vi "Update GEA FGV.vi"(8 "Error In":errorcluster, 10 "Enum":enum16{"Read", "Write"}(ring), 11 "GEA Inputs":T1 {"Destination" format="%.0x"; "Source" format="%.0x"}) -> (0 "Error Out":errorcluster, 3 "GEA Out":T1[](array[typedef]) {"Destination" format="%.0x"; "Source" format="%.0x"})   [LabVIEW 2016]
uses:
  Common/LabVIEW GEA2 Toolkit/LabVIEW_GEA2_Toolkit.lvlibp/type defs/Source_Destination.ctl
  Common/LabVIEW GEA2 Toolkit/LabVIEW_GEA2_Toolkit.lvlibp
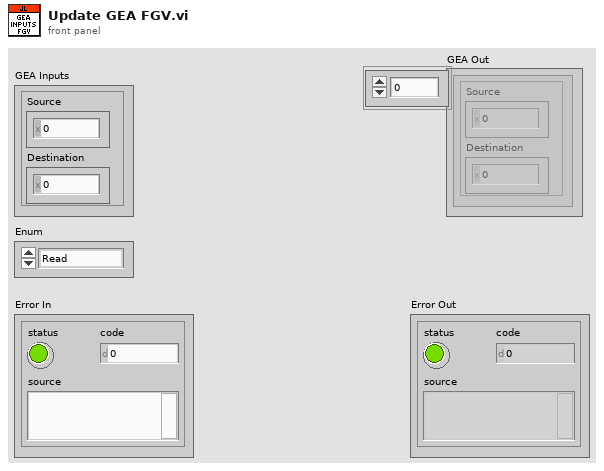
[diagram p1: front panel]
types:
  T1 = typedef "LabVIEW_GEA2_Toolkit.lvlibp/Source_Destination.ctl" = cluster{"Source":u8, "Destination":u8}
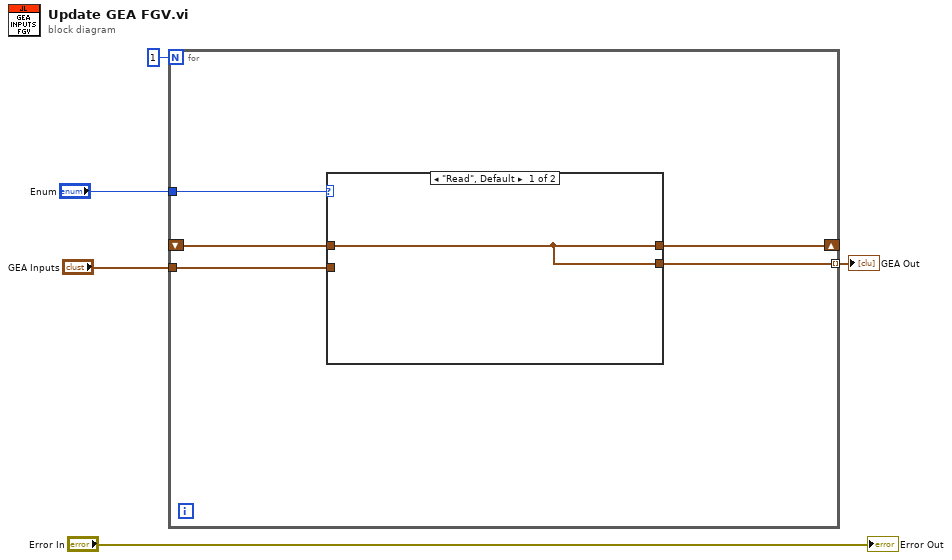
[diagram p0: block diagram]
diagram:
  n1 = for {
    N: 1 -> [_]
    shift-right: [w7] -> _
    shift-left: _ -> [w10]
    tunnel: "GEA Inputs" -> [w9]
    tunnel: "Enum" -> [w8]
    tunnel: [w6] -> w2 mode=indexing
    n2 = case shown="\"Read\", Default" w8 {
      tunnel: w10 -> [w11 _]
      tunnel: w9 -> [_ w12]
      tunnel: [w11 w12] -> w6
      tunnel: [w11 w12] -> w7
      frame "Read", Default {
      }
      frame "Write" {
      }
    }
  }
  "GEA Out" <- w2
  "Error Out" <- "Error In"
